vi "aStar.vi"(5 "endPos":cluster{"x":i32, "y":i32}={"x"=0, "y"=6}, 7 "curPos":cluster{"x":i32, "y":i32}, 11 "occupancy grid":dbl[][](array[numeric])) -> (3 "path":cluster{"X":i32, "Y":i32}[](array[cluster]))   [LabVIEW 2016]
uses:
  <vilib>/robotics/Navigation/shared/WorldMap/OccupancyGridWorldMap/NI_Robotics_OccupancyGridWorldMap.lvclass
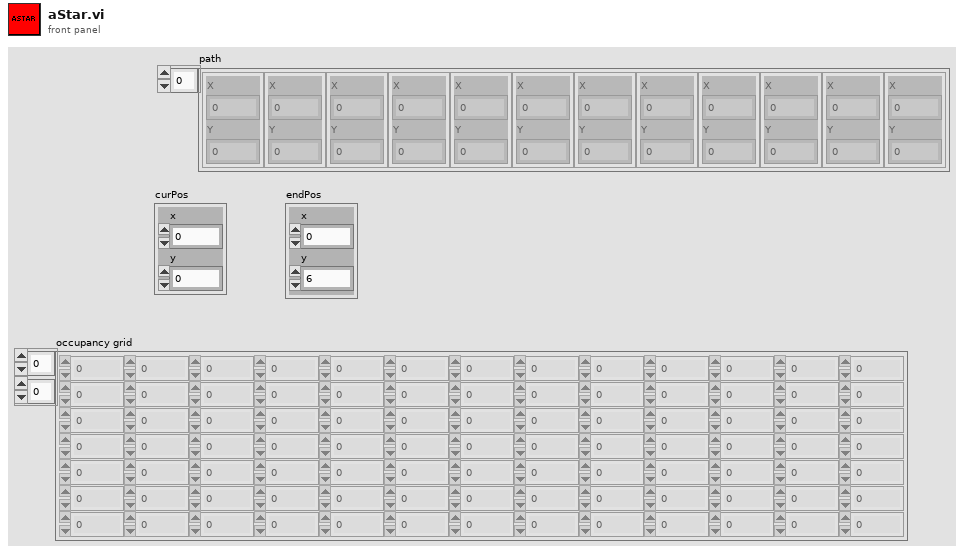
[diagram p1: front panel]
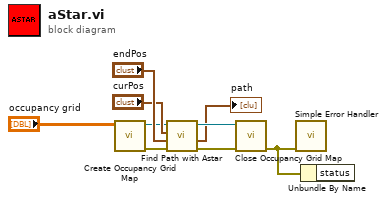
[diagram p0: block diagram]
diagram:
  n1 = call <vilib>:"Create Occupancy Grid Map.vi"("occupancy grid"="occupancy grid") -> ("error out"=w9:errorcluster, "map reference out"=w5:refnum<data-value>)  [unwired: 9 in]
  n2 = call "Find Path with Astar.vi"("error in (no error)"=w9, "goal node"="endPos", "start node"="curPos", "map reference in"=w5) -> ("error out"=w3:errorcluster, "Array"=→"path":cluster{"X":i32, "Y":i32}[], "map reference out"=w4:refnum<data-value>)  [unwired: 5 in]
  n3 = call <vilib>:"Close Occupancy Grid Map.vi"("error in (no error)"=w3, "map reference in"=w4) -> ("error out"=w2:errorcluster)  [unwired: 9 in]
  n4 = call <vilib>:"Simple Error Handler.vi"("error in (no error)"=w2) -> ()  [unwired: 4 in, 5 out]
  n5 = Unbundle By Name(w2) -> ()  [unwired: 1 out]
